vi "WS1050 36 DUT CP CV Sweep F12_B1_Ver1.2.vi"(0 "TMN DC\\CAP Data Log File Path":path=path "C:/WS1050 36 DUT Data", 1 "Test Program":string="WS1050 36 DUT CP CV Sweep SubVI", 3 "Lot#":string="WS1050", 4 "Wafer#":string="T7-EB", 5 "Board#":string="BRD5", 6 "Temp":string, 7 "error in (no error)":errorcluster, 8 "File Name":string="CYC_WS1050_T7_EB_65C_40V_25DC_EMPTY_BRD5_141017_1", 9 "Comment":string="CYC65C40V", 10 "Ke2400":refnum<visa-resource-name>="GPIB0::3::INSTR", 11 "PS1 Source":refnum<visa-resource-name>="GPIB0::5::INSTR", 12 "Serial Number":string[][](table)=[["DUT", "SN"], ["DUT1", "1"], ["DUT2", "2"], ["DUT3", "3"], ["DUT4", "4"], ["DUT5", "5"], ["DUT6", "6"], ["DUT7", "7"], ["DUT8", "8"], ["DUT9", "9"], ["DUT10", "10"], ["DUT11", "11"], ["DUT12", "12"], ["DUT13", "13"], ["DUT14", "14"], ["DUT15", "15"], ["DUT16", "16"], ["DUT17", "17"], ["DUT18", "18"], ["DUT19", "19"], ["DUT20", "20"], ["DUT21", "21"], ["DUT22", "22"], ["DUT23", "23"], ["DUT24", "24"], ["DUT25", "25"], ["DUT26", "26"], ["DUT27", "27"], ["DUT28", "28"], ["DUT29", "29"], ["DUT30", "30"], ["DUT31", "31"], ["DUT32", "32"], ["DUT33", "33"], ["DUT34", "34"], ["DUT35", "35"], ["DUT36", "36"]], 14 "CP Set to Run":dbl[][](array[numeric]), 16 "HD/Cycles Completed":string="Test Data", 18 "Ke2000":refnum<visa-resource-name>="GPIB0::9::INSTR") -> (13 "40V_1":string[][](table), 15 "40V_2":string[][](table), 17 "40V_3":string[][](table), 20 "Plot_1":dbl[][](graph) caption="(Y) Multi Plot 2", 21 "Plot_2":dbl[][](graph) caption="(Y) Multi Plot 2", 22 "Ke2400 Out":refnum<visa-resource-name>="GPIB0::3::INSTR", 23 "Plot_3":dbl[][](graph) caption="(Y) Multi Plot 2", 24 "CP Voltage":string, 25 "PS1 Out":refnum<visa-resource-name>, 26 "Ke2000 Out":refnum<visa-resource-name>="GPIB0::9::INSTR", 27 "error out":errorcluster)   [LabVIEW 2012]
uses:
  WS_VCAP Driver 029/Source/WSVCAP Shell/Type Defs/WSVCAP SHL I2C DUT Mask Mode Enum.ctl
panel:
  in  "Reg1_Bit Cntrl":string[](array[string])=["01", "02", "04", "08", "10", "20", "40", "80", "03", "06", "0C", "D8", "33", "66", "CC", "07", "0E", "1C", "38", "70", "E0", "0F", "1E", "3C", "78", "F0", "1F", "3E", "7C", "F8", "3F", "7E", "FC", "7F", "FE", "FD", "FB", "F7", "EF", "DF", "BF", "7F", "FC", "F9", "F3", "E7", "CF", "9F", "3F", "F8", "F1", "E3", "C7", "8F", "1F", "F0", "E1", "C3", "87", "0F", "E0", "C1", "83", "07", "C0", "81", "03", "AA", "55", "00"]
  out "date string":string="5/19/2014"
  in  "VPI_Cmd":string[](array[string])=["00", "3B", "00"]
  in  "VPI Name":string[](array[string])=["All_Drivers OFF", "All Drivers ON", "All Drivers OFF2"]
  in  "Tab Control":T1(tab)
  in  "Set VDD":dbl=3.7 format="%.3g"
  in  "Clock Rate (Hz)":dbl=1000000.0 caption="Meas Speed" format="%.1p Hz"
  out "AR  Measurent(Hz)":dbl
  in  "RFFE Slave Address":u8=7 caption="Slave Address" format="0x%02x"
  in  "CP VPI":i32(ring) items=["CP HDC 35V", "CP HDC 40.25V", "CP HDC 27.5V", "CP HDC 30.5V", "CP HDC 44V"]
  in  "Control Panel":T2={"CP C-V \nSweep"=TRUE, "HD/CYC"=FALSE, "E-CAL"=FALSE, "DVA"=FALSE, "VPI"=FALSE, "VSA"=FALSE, "HS"=FALSE}
  out "CP C-V Sweep":bool
  out "HD/CYC":bool
  out "E-CAL":bool
  out "DVA":bool
  out "VPI":bool
  out "VSA":bool
  out "HS":bool
  in  "Freq(Hz)":string="12K"
  in  "Test Sequences":i32(ring) items=["C1_C2_C3", "C2_C1_C3", "C3_C2_C1"]
  in  "WS1050/51":bool=TRUE
  in  "CP with DVA ON":i32(ring) items=["CP HDC 35V", "CP HDC 40.25V", "CP HDC 27.5V", "CP HDC 30.5V", "CP HDC 44V"]
  in  "% Duty Cycle":string="NA"
  in  "Cmin/Act":bool=TRUE
  in  "Current Input":string="71.772763E+0"
  out "NOM IDD OFF(uA)":string
  out "No of HD/Cycle\nCompleted":i32
  out "Loop \ncompleted":i32=1
  out "Previous Time":string="12:20:26 PM"
  out "STATUS":string="Idle...."
  out "Total Delta C2(pF)":string[](array[string])
  out "Total Delta C1(pF)":string[](array[string])
  out "Total Delta C3(pF)":string[](array[string])
  out "VPI C2":string[][](table)
  out "VPI C3":string[][](table)
  out "NOM IDD ON (uA)":string
  out "IDD_HD/CYC (uA)":string="164.601255E+0"
  out "IDD Stdby(uA)":string="2.606990E+0"
  out "VPI C1":string[][](table)
  out "Loops Run":i64
  out "VSA_V1":string[][](table)
  out "VSA_V2":string[][](table)
  out "VSA_V3":string[][](table)
  in  "VSA Voltage(V)":dbl[](array[numeric])=[-10.0, 0.0, 10.0]
  in  "X Repeat":i32=100
  out "% Delta C_T0":string[][](array[string])
  out "% Delta C":string[][](array[string])
  out "EFuse RB T0":string[](array[string])
  out "Current EFuse Read back":string[](array[string])
  out "EFuse Readback Status":bool[](array[boolean])
  in  "DeltaC Target Setting(pF)":dbl=7.375
  in  "Debug":bool
  in  "No of Rows\nFrom Spread Sheet":i32
  in  "Plot Delta Cmin":bool=TRUE
  in  "Plot":T3(ring)
  in  "Bank1":i32(ring)=6 items=["C1", "C2", "C3", "D_C1", "D_C2", "D_C3", "D_B1_C1", "D_B1_C2", "D_B1_C3"]
  in  "Bank2":i32(ring)=7 items=["C1", "C2", "C3", "D_C1", "D_C2", "D_C3", "D_B1_C1", "D_B1_C2", "D_B1_C3"]
  in  "Bank3":i32(ring)=8 items=["C1", "C2", "C3", "D_C1", "D_C2", "D_C3", "D_B1_C1", "D_B1_C2", "D_B1_C3"]
  # "Company:  WiSpry Inc\n20 Fairbanks Ste 198 Irvine CA 92618\n\nAuthor:  Andy V Tran\nCreated:  08/21/2015\nLabVIEW 2012 Pro\nTest Program:  WS1050 36 DUT CP CV Sweep SubVI\nFPGA: WS_VCAP Driver 029"
  # "Note for HD Duty Cycle:\n1.  Set time to start HD_DC (Min), default is 259200 (6 months) \n2.  Set Time for Duty Cycle ON/OFF, default setting is 2 minutes\n3.  No of Loops to RP = 3600s/(Time ALL ON(s) + Time ALL + OFF(s))\n4.  Set X Repeat = no of runs, default is 100 runs\n5.  Set TTF Completed to stop the test.\n\nVer 1.1 updated based on Ver1.0:\n1.  Updated the control panel ( CP C-V Sweep was set \"Yes\" by default)\n2.  CP Voltage sweep should be set up from look up table."
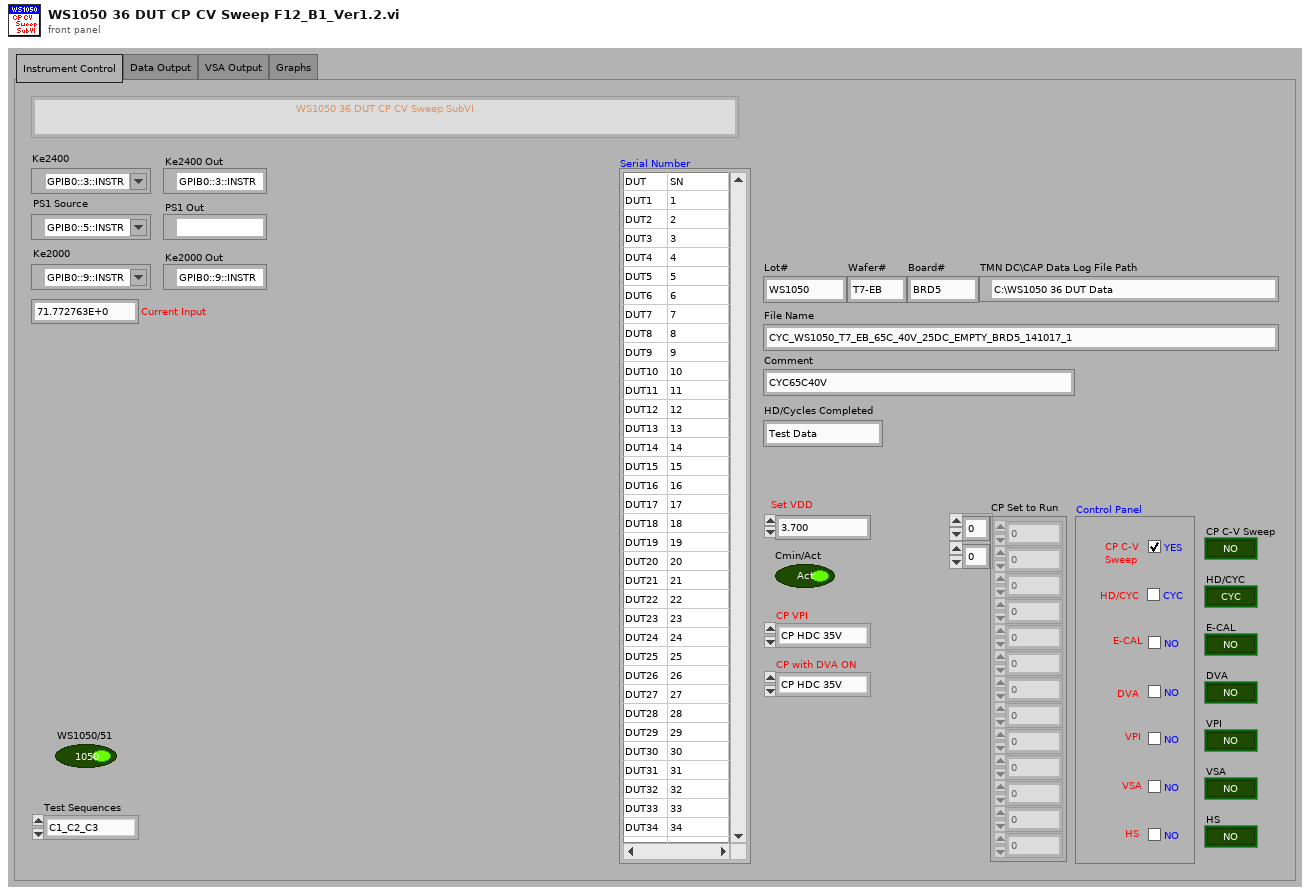
[diagram p1: front panel]
types:
  T1 = enum32{"Instrument Control", "Data Output", "VSA Output", "Graphs"}
  T2 = cluster{"CP C-V \nSweep":bool, "HD/CYC":bool, "E-CAL":bool, "DVA":bool, "VPI":bool, "VSA":bool, "HS":bool}
  T3 = enum16{"ALL DUTs", "DUT 01", "DUT 02", "DUT 03", "DUT 04", "DUT 05", "DUT 06", "DUT 07", "DUT 08", "DUT 09", "DUT 10", "DUT 11", "DUT 12", "DUT 13", "DUT 14", "DUT 15", "DUT 16", "DUT 17", "DUT 18", "DUT 19", "DUT 20", "DUT 21", "DUT 22", "DUT 23", "DUT 24", "DUT 25", "DUT 26", "DUT 27", "DUT 28", "DUT 29", "DUT 30", "DUT 31", "DUT 32", "DUT 33", "DUT 34", "DUT 35", "DUT 36"}
  T4 = typedef "WSVCAP SHL I2C DUT Mask Mode Enum.ctl" = enum16{"Custom", "C1", "C2", "C3", "All"}
  T5 = cluster{"Test Program ":string, "Comment":string, "Data Out":string, "Data Out":string, "CP Voltage":string, string, "% Duty Cycle":string, "CP Voltage":string, "string":string, "Freq(Hz)":string, "Board#":string}
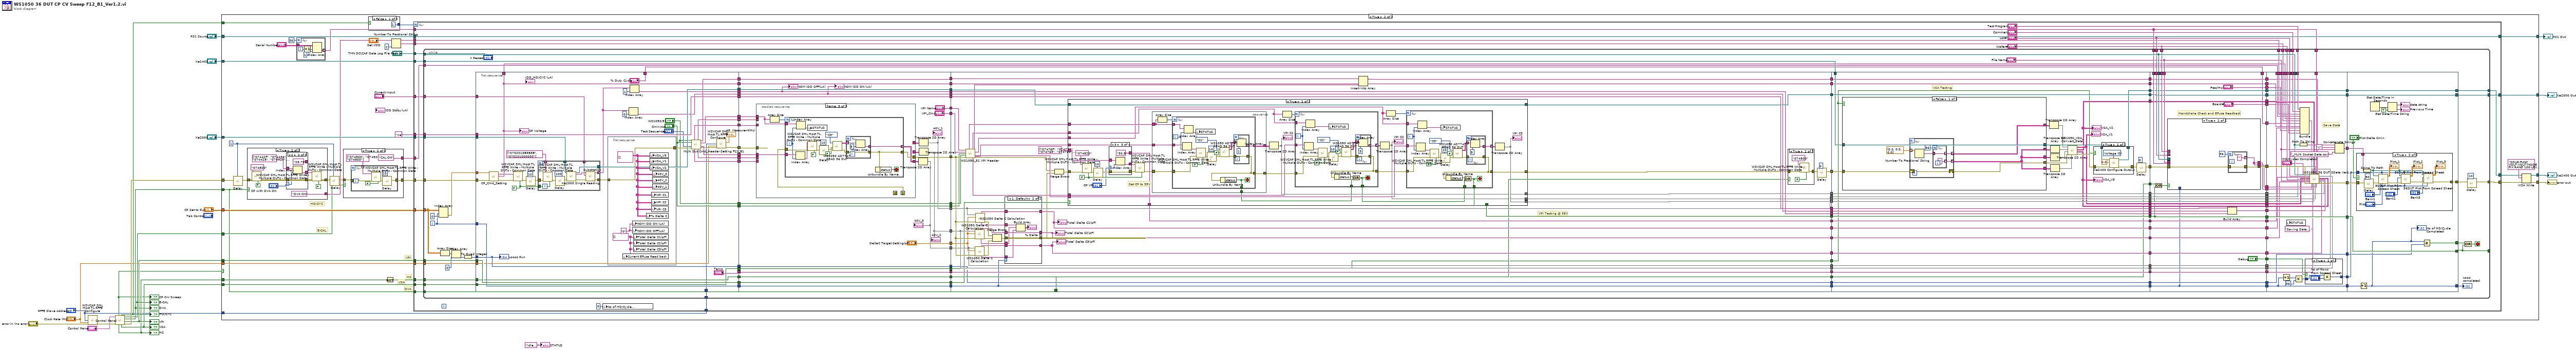
[diagram p0: block diagram]
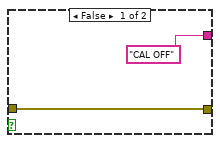
[diagram p3: hidden frame]
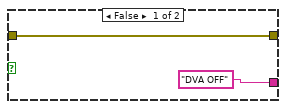
[diagram p4: hidden frame]
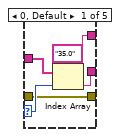
[diagram p5: hidden frame]
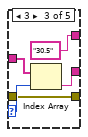
[diagram p6: hidden frame]
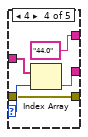
[diagram p7: hidden frame]
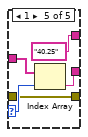
[diagram p8: hidden frame]
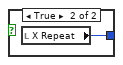
[diagram p9: hidden frame]
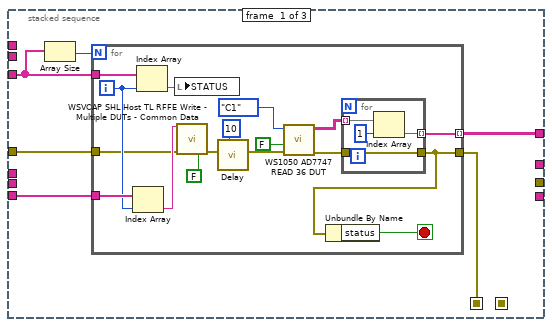
[diagram p10: hidden frame]
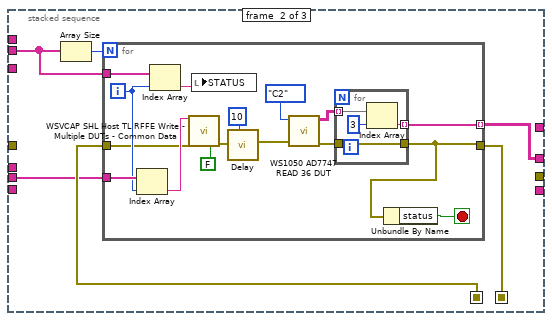
[diagram p11: hidden frame]
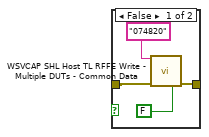
[diagram p12: hidden frame]
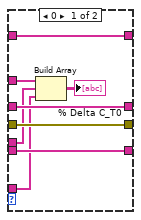
[diagram p13: hidden frame]
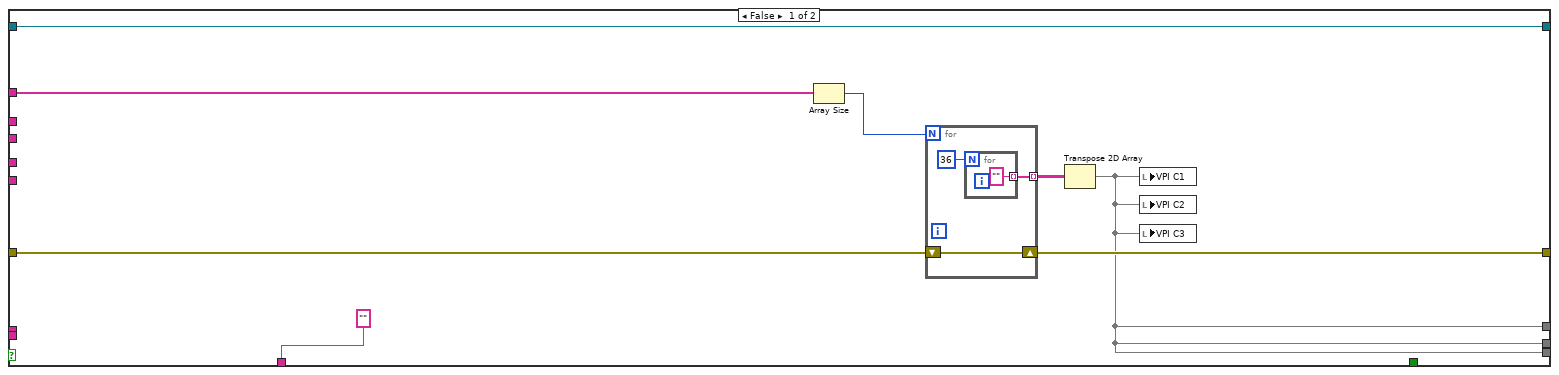
[diagram p14: hidden frame]
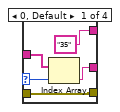
[diagram p15: hidden frame]
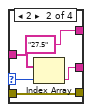
[diagram p16: hidden frame]
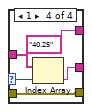
[diagram p17: hidden frame]
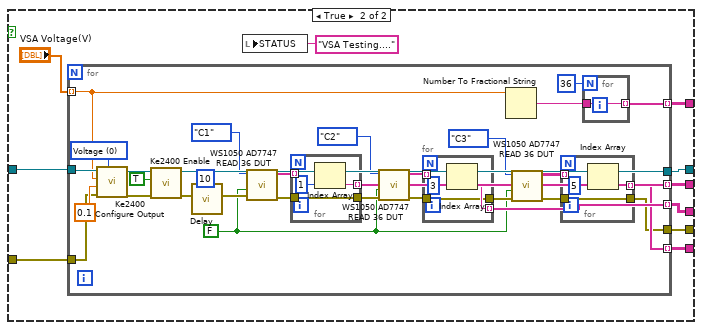
[diagram p19: hidden frame]
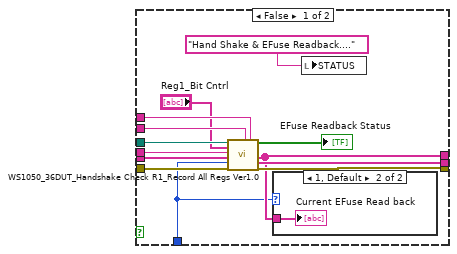
[diagram p20: hidden frame]
diagram:
  n1 = call "WSVCAP SHL Host TL RFFE Configure.vi"("RFFE Slave Address"="RFFE Slave Address", "Clock Rate (Hz)"="Clock Rate (Hz)", "error in"="error in (no error)") -> ("error out"=w4:errorcluster)  [unwired: 11 in, 1 out]
  n2 = call "Control Panel.vi"("error in (no error)"=w4, "Control Panel"="Control Panel") -> ("error out"=w12:errorcluster, "VPI"=w8:bool, "DVA"=w9:bool, "E-CAL"=w10:bool, "VSA"=w7:bool, "HD/CYC"=w11:bool, "HS"=w6:bool, "Verify Socket"=w1:bool)  [unwired: 2 in]
  "CP C-V Sweep" <- w1
  "E-CAL" <- w10
  "VPI" <- w8
  "VSA" <- w7
  "HS" <- w6
  "HD/CYC" <- w11
  "DVA" <- w9
  n3 = case shown="True" w1 {
    tunnel: w12 -> [w26 w29]
    tunnel: [w26 w34] -> w15
    tunnel: "CP Set to Run" -> [_ w64]
    tunnel: "PS1 Source" -> [w24 w31]
    tunnel: "Ke2000" -> [w25 w28]
    tunnel: [w25 w63] -> w22
    tunnel: [w24 w35] -> w21
    tunnel: "Ke2400" -> [w23 w61]
    tunnel: [w23 w58] -> w16
    tunnel: "RFFE Slave Address" -> [_ w56]
    tunnel: w11 -> [_ w41]
    tunnel: w10 -> [_ w40]
    tunnel: w9 -> [_ w30]
    tunnel: w8 -> [_ w39]
    tunnel: w7 -> [_ w38]
    tunnel: w6 -> [_ w37]
    tunnel: "Clock Rate (Hz)" -> [_ w33]
    frame False {
    }
    frame True {
      w32 = u32 1 ("milliseconds to wait")
      # "VSA"
      # "HS"
      # "HD/CYC"
      # "DVA"
      # "E-CAL"
      # "VPI"
      n4 = call "Delay.vi"("milliseconds to wait"=w32, "error in (no error)"=w29) -> ("error out"=w55:errorcluster)  [unwired: 9 in]
      n5 = case shown="True" w30 {
        tunnel: w55 -> [w82 w92]
        tunnel: [w82 w90] -> w53
        tunnel: ["DVA OFF" ("Data Out") "DVA ON" ("Data Out")] -> w54
        frame False {
        }
        frame True {
          n6 = call "WSVCAP SHL Host TL RFFE Write - Multiple DUTs - Common Data.vi"("Data Out"="074800", "error in"=w92, "Log (T)"=FALSE) -> ("error out"=w88:errorcluster)  [unwired: 12 in]
          n7 = case shown="2" "CP with DVA ON" {
            selector: "CP with DVA ON" -> [w98 w103 w108 w113 w117]
            tunnel: string[] ["07442F", "074436", "074428", "074429", "07443B"] -> [w99 w104 w109 w114 w119]
            tunnel: [w97 w102 w107 w112 w118] -> w84
            tunnel: ["35.0" ("Data Out") "29.75" ("Data Out") "30.5" ("Data Out") "44.0" ("Data Out") "40.25" ("Data Out")] -> _
            tunnel: w88 -> [w95 w100 w105 w110 w115]
            tunnel: [w95 w100 w105 w110 w115] -> w87
            frame 0, Default {
              n8 = Index Array(array=w99, index=w98) -> (element=w97:string)
            }
            frame 2 {
              n9 = Index Array(array=w104, index=w103) -> (element=w102:string)
            }
            frame 3 {
              n10 = Index Array(array=w109, index=w108) -> (element=w107:string)
            }
            frame 4 {
              n11 = Index Array(array=w114, index=w113) -> (element=w112:string)
            }
            frame 1 {
              n12 = Index Array(array=w119, index=w117) -> (element=w118:string)
            }
          }
          n13 = call "WSVCAP SHL Host TL RFFE Write - Multiple DUTs - Common Data.vi"("Data Out"=w84, "error in"=w87, "Log (T)"=FALSE) -> ("error out"=w90:errorcluster)  [unwired: 12 in]
        }
      }
      n14 = for {
        N: 36 -> [_]
        tunnel: "Serial Number" -> [w69]
        tunnel: [w67] -> w43 mode=indexing
        i -> [w66]
        n15 = Increment(x=w66) -> (x+1=w65:i32)
        n16 = Index Array(array=w69, index (row)=w65, index (col)=1 ("disabled index (col)")) -> (element=w67:string)
      }
      n17 = call "Delay.vi"("milliseconds to wait"=w32, "error in (no error)"=w53) -> ("error out"=w48:errorcluster)  [unwired: 9 in]
      n18 = case shown="True" w40 {
        tunnel: w48 -> [w70 w73]
        tunnel: [w70 w72] -> w47
        tunnel: ["CAL OFF" ("Data Out") "CAL ON" ("Data Out")] -> w49
        frame False {
        }
        frame True {
          n19 = for {
            tunnel: string[] ["074900", "074920", "074900"] -> [w81] mode=indexing
            tunnel: w73 -> [w78]
            tunnel: [w77] -> w72
            n20 = call "WSVCAP SHL Host TL RFFE Write - Multiple DUTs - Common Data.vi"("Data Out"=w81, "error in"=w78, "Log (T)"=FALSE) -> ("error out"=w80:errorcluster)  [unwired: 12 in]
            n21 = call "Delay.vi"("milliseconds to wait"=u32 10, "error in (no error)"=w80) -> ("error out"=w77:errorcluster)  [unwired: 9 in]
          }
        }
      }
      n22 = case shown="False" w41 {
        tunnel: [1 ("X Repeat") w121] -> w57
        frame False {
        }
        frame True {
          n23 = local read "X Repeat"() -> (w121:i32)
        }
      }
      n24 = Not(x=w37) -> (.not. x?=w42:bool)
      n25 = Number To Fractional String(number="Set VDD", precision (6)=i16 2) -> (F-format string=w51:string)  [unwired: 2 in]
      n26 = for {
        N: w57 -> [_]
        tunnel: w64 -> [w147]
        tunnel: [w143] -> w63
        tunnel: "na" ("In1 - In2") -> [w142]
        tunnel: w28 -> [w141]
        tunnel: "TMN DC\\CAP Data Log File Path" -> [w140]
        tunnel: w61 -> [w138]
        tunnel: [w137] -> w59
        tunnel: w31 -> [w124]
        tunnel: w56 -> [w135]
        tunnel: w54 -> [w134]
        tunnel: w51 -> [w133]
        tunnel: [w132] -> w50
        tunnel: w49 -> [w131]
        tunnel: w47 -> [w130]
        tunnel: w30 -> [w129]
        tunnel: w39 -> [w128]
        tunnel: w42 -> [w127]
        tunnel: w38 -> [w126]
        tunnel: w43 -> [w125]
        tunnel: [w124] -> w35
        tunnel: "Current Input" -> [w123]
        tunnel: w33 -> [w122]
        n27 = while {
          tunnel: w147 -> [w171]
          tunnel: w140 -> [w318]
          tunnel: "Lot#" -> [w317]
          tunnel: "Wafer#" -> [w316]
          tunnel: w125 -> [w315]
          tunnel: "Test Program" -> [w314]
          tunnel: w125 -> [w313]
          tunnel: "Comment" -> [w312]
          tunnel: "Lot#" -> [w311]
          tunnel: "Wafer#" -> [w310]
          tunnel: w141 -> [w307]
          tunnel: [w309] -> w143
          tunnel: w142 -> [w306]
          tunnel: w138 -> [w304]
          tunnel: [w303] -> w137
          tunnel: [w228] -> _
          tunnel: w135 -> [w227]
          tunnel: w134 -> [w210]
          tunnel: w133 -> [w209]
          tunnel: [w194] -> w132
          tunnel: w131 -> [w198]
          tunnel: w130 -> [w154]
          tunnel: w129 -> [w197]
          tunnel: w128 -> [w191]
          tunnel: w127 -> [w188]
          tunnel: w126 -> [w184]
          tunnel: w123 -> [w159]
          tunnel: w122 -> [w158]
          i -> [w172]
          stop <- w257 stop-if-true
          n28 = Index Array(array=w171, index (row)=w172, index (col)=0 ("disabled index (col)")) -> (element=w168:dbl)
          n29 = Array Size(array=w171) -> (size(s)=w170:i32[])
          n30 = Index Array(array=w170, index=0) -> (element=w161:i32)
          n31 = To Quad Integer(1:w161) -> (0:w160:i64)
          n32 = flat-sequence {
            tunnel: [w360] -> w302
            tunnel: w307 -> [w327]
            tunnel: w306 -> [w361]
            tunnel: [w361] -> w301
            tunnel: [w343] -> w300
            tunnel: [w340] -> w299
            tunnel: w154 -> [w326]
            tunnel: w172 -> [w328]
            tunnel: [w328] -> w256
            tunnel: ["Temp"] -> w251
            tunnel: [w347] -> w246
            tunnel: [w346] -> w245
            tunnel: [w345] -> w244
            tunnel: [w351] -> w234
            tunnel: [w348] -> w233
            tunnel: w227 -> [w319]
            tunnel: [w350] -> w218
            tunnel: [w349] -> w217
            tunnel: ["% Duty Cycle"] -> w208
            tunnel: [w325] -> w202
            tunnel: w191 -> [w357]
            tunnel: [w357] -> w190
            tunnel: w188 -> [w356]
            tunnel: [w356] -> w187
            tunnel: w184 -> [w355]
            tunnel: [w355] -> w183
            tunnel: [w322] -> w180
            tunnel: ["WS1050/51"] -> w177
            tunnel: ["Cmin/Act"] -> w175
            tunnel: w160 -> [w332]
            tunnel: w168 -> [w333]
            tunnel: [w332] -> w167
            tunnel: w159 -> [w331]
            tunnel: w158 -> [w320]
            tunnel: [w325] -> w155
            tunnel: w302 -> [w406]
            tunnel: w301 -> [w409]
            tunnel: w300 -> [w405]
            tunnel: w299 -> [w404]
            tunnel: [w399] -> w226
            tunnel: [w409] -> w225
            tunnel: [w405] -> w224
            tunnel: [w404] -> w223
            tunnel: w256 -> [w408]
            tunnel: [w408] -> w222
            tunnel: w251 -> [w407]
            tunnel: [w407] -> w221
            tunnel: [w406] -> w220
            tunnel: w246 -> [w403]
            tunnel: w245 -> [w386]
            tunnel: w244 -> [w387]
            tunnel: [w401] -> w219
            tunnel: w234 -> [w402]
            tunnel: w233 -> [w401]
            tunnel: w218 -> [w390]
            tunnel: w217 -> [w385]
            tunnel: [w400] -> w203
            tunnel: w202 -> [w400]
            tunnel: w190 -> [w398]
            tunnel: [w398] -> w189
            tunnel: w187 -> [w397]
            tunnel: [w397] -> w186
            tunnel: w183 -> [w396]
            tunnel: [w396] -> w182
            tunnel: w180 -> [w391]
            tunnel: w177 -> [w394]
            tunnel: [w394] -> w176
            tunnel: w175 -> [w393]
            tunnel: [w393] -> w174
            tunnel: w167 -> [w392]
            tunnel: [w392] -> w166
            tunnel: [w388] -> w153
            tunnel: [w384] -> w152
            tunnel: [w382] -> w151
            tunnel: ["DeltaC Target Setting(pF)"] -> w150
            tunnel: ["VPI Name"] -> w149
            tunnel: ["VPI_Cmd"] -> w148
            tunnel: [w544] -> w298
            tunnel: [w513] -> w297
            tunnel: [w533] -> w296
            tunnel: [w524] -> w295
            tunnel: [w546] -> w294
            tunnel: [w545] -> w293
            tunnel: [w543] -> w292
            tunnel: [w539] -> w291
            tunnel: [w538] -> w290
            tunnel: [w534] -> w255
            tunnel: [w542] -> w250
            tunnel: [w540] -> w247
            tunnel: [w537] -> w243
            tunnel: [w535] -> w242
            tunnel: [w532] -> w237
            tunnel: [w521] -> w232
            tunnel: [w520] -> w231
            tunnel: [w519] -> w230
            tunnel: [w518] -> w204
            tunnel: [w517] -> w201
            tunnel: [w510] -> w185
            tunnel: [w509] -> w181
            tunnel: [w496] -> w165
            tunnel: w150 -> [w530]
            tunnel: w151 -> [w524]
            tunnel: w152 -> [w531]
            tunnel: w226 -> [w533]
            tunnel: w225 -> [w543]
            tunnel: w224 -> [w539]
            tunnel: w223 -> [w538]
            tunnel: w222 -> [w534]
            tunnel: w221 -> [w542]
            tunnel: w220 -> [w541]
            tunnel: w219 -> [w536]
            tunnel: w203 -> [w518]
            tunnel: w189 -> [w511]
            tunnel: w186 -> [w510]
            tunnel: w182 -> [w509]
            tunnel: w176 -> [w508]
            tunnel: w174 -> [w497]
            tunnel: w166 -> [w496]
            tunnel: w153 -> [w532]
            tunnel: w197 -> [w516]
            tunnel: w149 -> [w492]
            tunnel: w148 -> [w491]
            tunnel: w298 -> [w751]
            tunnel: [w751] -> w289
            tunnel: [w737] -> w288
            tunnel: [w750] -> w287
            tunnel: w297 -> [w749]
            tunnel: w296 -> [w748]
            tunnel: w295 -> [w747]
            tunnel: [w748] -> w286
            tunnel: [w747] -> w285
            tunnel: w294 -> [w746]
            tunnel: [w746] -> w284
            tunnel: w293 -> [w745]
            tunnel: [w745] -> w283
            tunnel: w292 -> [w744]
            tunnel: [w744] -> w282
            tunnel: w291 -> [w743]
            tunnel: [w743] -> w281
            tunnel: w290 -> [w742]
            tunnel: [w742] -> w280
            tunnel: w304 -> [w741]
            tunnel: [w739] -> w279
            tunnel: [w719] -> w278
            tunnel: [w720] -> w277
            tunnel: [w718] -> w276
            tunnel: w255 -> [w735]
            tunnel: [w735] -> w254
            tunnel: w250 -> [w734]
            tunnel: [w734] -> w249
            tunnel: w247 -> [w750]
            tunnel: w243 -> [w732]
            tunnel: w242 -> [w733]
            tunnel: [w733] -> w241
            tunnel: [w732] -> w239
            tunnel: w237 -> [w731]
            tunnel: [w731] -> w236
            tunnel: w232 -> [w717]
            tunnel: w231 -> [w716]
            tunnel: w230 -> [w715]
            tunnel: [w712] -> w229
            tunnel: [w717] -> w216
            tunnel: [w716] -> w214
            tunnel: [w715] -> w212
            tunnel: [w714] -> w205
            tunnel: w204 -> [w714]
            tunnel: w201 -> [w713]
            tunnel: [w713] -> w200
            tunnel: w185 -> [w712]
            tunnel: w181 -> [w711]
            tunnel: w165 -> [w710]
            tunnel: [w710] -> w164
            tunnel: w289 -> [w845]
            tunnel: [w845] -> w275
            tunnel: w288 -> [w866]
            tunnel: [w865] -> w274
            tunnel: w318 -> [w867]
            tunnel: w317 -> [w864]
            tunnel: w316 -> [w863]
            tunnel: w315 -> [w862]
            tunnel: [w861] -> w273
            tunnel: w287 -> [w855]
            tunnel: [w855] -> w272
            tunnel: w286 -> [w860]
            tunnel: w285 -> [w859]
            tunnel: [w860] -> w271
            tunnel: [w859] -> w270
            tunnel: [w853] -> w269
            tunnel: w284 -> [w858]
            tunnel: [w858] -> w268
            tunnel: w283 -> [w857]
            tunnel: [w857] -> w267
            tunnel: [w856] -> w266
            tunnel: w282 -> [w854]
            tunnel: w281 -> [w852]
            tunnel: w280 -> [w851]
            tunnel: "File Name" -> [w850]
            tunnel: w279 -> [w849]
            tunnel: [w849] -> w265
            tunnel: w278 -> [w848]
            tunnel: [w848] -> w264
            tunnel: [w847] -> w263
            tunnel: w277 -> [w847]
            tunnel: w276 -> [w846]
            tunnel: [w846] -> w262
            tunnel: w254 -> [w829]
            tunnel: [w829] -> w252
            tunnel: w249 -> [w843]
            tunnel: [w843] -> w248
            tunnel: w241 -> [w842]
            tunnel: [w842] -> w240
            tunnel: w239 -> [w841]
            tunnel: [w841] -> w238
            tunnel: w236 -> [w840]
            tunnel: [w840] -> w235
            tunnel: w229 -> [w839]
            tunnel: w216 -> [w838]
            tunnel: [w838] -> w215
            tunnel: w214 -> [w837]
            tunnel: [w837] -> w213
            tunnel: w212 -> [w836]
            tunnel: [w836] -> w211
            tunnel: w208 -> [w835]
            tunnel: [w835] -> w207
            tunnel: [w834] -> w206
            tunnel: w205 -> [w834]
            tunnel: w200 -> [w833]
            tunnel: [w833] -> w199
            tunnel: ["Freq(Hz)"] -> w179
            tunnel: ["Board#"] -> w178
            tunnel: w164 -> [w830]
            tunnel: [w830] -> w163
            tunnel: ["Debug"] -> w157
            tunnel: w275 -> [w940]
            tunnel: w274 -> [w939]
            tunnel: w318 -> [w906]
            tunnel: w314 -> [w934]
            tunnel: w313 -> [w937]
            tunnel: w312 -> [w933]
            tunnel: w311 -> [w936]
            tunnel: w310 -> [w932]
            tunnel: w273 -> [w935]
            tunnel: [w940] -> w259
            tunnel: [w938] -> w260
            tunnel: w272 -> [w930]
            tunnel: [w930] -> w261
            tunnel: w271 -> [w929]
            tunnel: w270 -> [w917]
            tunnel: w269 -> [w928]
            tunnel: w268 -> [w927]
            tunnel: w267 -> [w919]
            tunnel: w266 -> [w926]
            tunnel: "File Name" -> [w900]
            tunnel: w265 -> [w925]
            tunnel: [w925] -> w258
            tunnel: w264 -> [w924]
            tunnel: w263 -> [w923]
            tunnel: w262 -> [w922]
            tunnel: [w902] -> w253
            tunnel: w252 -> [w902]
            tunnel: w248 -> [w921]
            tunnel: w240 -> [w920]
            tunnel: w238 -> [w918]
            tunnel: w235 -> [w889]
            tunnel: w215 -> [w916]
            tunnel: w213 -> [w915]
            tunnel: w211 -> [w914]
            tunnel: w210 -> [w913]
            tunnel: w198 -> [w912]
            tunnel: w155 -> [w911]
            tunnel: w209 -> [w910]
            tunnel: w207 -> [w909]
            tunnel: w206 -> [w908]
            tunnel: w199 -> [w907]
            tunnel: [w904] -> w196
            tunnel: [w897] -> w192
            tunnel: w179 -> [w896]
            tunnel: w178 -> [w894]
            tunnel: w163 -> [w893]
            tunnel: [w893] -> w162
            tunnel: w157 -> [w891]
            tunnel: [w958] -> w308
            tunnel: [w959] -> w309
            tunnel: [w960] -> w228
            tunnel: w261 -> [w959]
            tunnel: w260 -> [w952]
            tunnel: w259 -> [w960]
            tunnel: w258 -> [w953]
            tunnel: [w953] -> w303
            tunnel: w253 -> [w946]
            tunnel: [w951] -> w193
            tunnel: w196 -> [w950]
            tunnel: w192 -> [w948]
            tunnel: w162 -> [w947]
            tunnel: [w945] -> w156
            frame #0 {
              w354 = FALSE ("Log (T)")
              n33 = call "CP_Cmd_Setting.vi"("error in (no error)"=w326, "Input"=w333) -> ("error out"=w335:errorcluster, "CP Voltage"=w325:string, "Send Cmd"=w334:string)  [unwired: 6 in, 1 out]
              "CP Voltage" <- w325
              n34 = call "WSVCAP SHL Host TL RFFE Write - Multiple DUTs - Common Data.vi"("Data Out"=w334, "error in"=w335, "Log (T)"=w354) -> ("error out"=w358:errorcluster)  [unwired: 12 in]
              n35 = call "Delay.vi"("milliseconds to wait"=u32 10, "error in (no error)"=w358) -> ("error out"=w338:errorcluster)  [unwired: 9 in]
              n36 = for {
                tunnel: [w374] -> w360
                tunnel: [w373] -> w324
                tunnel: w354 -> [w372]
                tunnel: w327 -> [w371]
                tunnel: w338 -> [w367]
                tunnel: string[] ["0702013B3B3B", "070201000000"] -> [w364] mode=indexing
                tunnel: [w363] -> w341 mode=indexing
                tunnel: w331 -> [w362]
                n37 = call "WSVCAP SHL Host TL RFFE Write - Multiple DUTs - Common Data.vi"("Data Out"=w364, "error in"=w367, "Log (T)"=w372) -> ("error out"=w368:errorcluster)  [unwired: 12 in]
                n38 = call "Delay.vi"("milliseconds to wait"=u32 100, "error in (no error)"=w368) -> ("error out"=w369:errorcluster)  [unwired: 9 in]
                n39 = call "Ke2000 Single Reading.vi"("error in (no error)"=w369, "VISA resource name"=w371) -> ("error out"=w366:errorcluster, "VISA resource name out"=w374:refnum<visa-resource-name>, "uA"=w365:string)  [unwired: 5 in, 2 out]
                n40 = call "Substration.vi"("error in (no error)"=w366, "Input2"=w362, "Input1"=w365) -> ("error out"=w373:errorcluster, "In1 - In2"=w363:string)  [unwired: 7 in]
              }
              n41 = flat-sequence {
                tunnel: [w375] -> w353
                tunnel: w324 -> [w375]
                frame #0 {
                  w376 = "0" ("NOM IDD OFF(uA)")
                  w377 = string[] []
                  w378 = string[][] []
                  n42 = local write "Current EFuse Read back"(w377) -> ()
                  n43 = local write "NOM IDD ON (uA)"(w376) -> ()
                  n44 = local write "NOM IDD OFF(uA)"(w376) -> ()
                  n45 = local write "Total Delta C1(pF)"(w377) -> ()
                  n46 = local write "Total Delta C2(pF)"(w377) -> ()
                  n47 = local write "Total Delta C3(pF)"(w377) -> ()
                  n48 = local write "% Delta C"(w378) -> ()
                  n49 = local write "VSA_V3"(w378) -> ()
                  n50 = local write "VSA_V1"(w378) -> ()
                  n51 = local write "VSA_V2"(w378) -> ()
                  n52 = local write "VPI C1"(w378) -> ()
                  n53 = local write "VPI C2"(w378) -> ()
                  n54 = local write "VPI C3"(w378) -> ()
                  n55 = local write "40V_3"(w378) -> ()
                  n56 = local write "40V_2"(w378) -> ()
                  n57 = local write "40V_1"(w378) -> ()
                }
              }
              n58 = Index Array(array=w341, index=0) -> (element=w343:string)
              n59 = Index Array(array=w341, index=1) -> (element=w340:string)
              n60 = call "Multi Dut Cmd_Header Setting F12_B1.vi"("WS1050/51"="WS1050/51", "Cmin/Act"="Cmin/Act", "Test Seq"="Test Sequences", "error in (no error)"=w353) -> ("Name 1"=w351:string[], "Name 2"=w350:string[], "Name Header"=w348:string[], "Name 3"=w349:string[], "Cmd 3"=w345:string[], "Cmd 1"=w347:string[], "Cmd 2"=w346:string[], "error out"=w321:errorcluster)  [unwired: 2 in, 2 out]
              n61 = call "WSVCAP SHL Host TL RFFE Configure.vi"("RFFE Slave Address"=w319, "Clock Rate (Hz)"=w320, "error in"=w321) -> ("Actual Rate (Hz)"=→"AR  Measurent(Hz)":dbl, "error out"=w322:errorcluster)  [unwired: 11 in]
              "Loops Run" <- w332
            }
            frame #1 {
              n62 = stacked-sequence {
                seq-local: [w410 _ _] -> [_ w442 _]
                seq-local: [_ w439 _] -> [_ _ w468]
                tunnel: w403 -> [w415 _ _]
                tunnel: w402 -> [w411 _ _]
                tunnel: w391 -> [w414 _ _]
                tunnel: [w413 _ _] -> w395
                tunnel: w390 -> [_ w440 _]
                tunnel: [_ w438 _] -> w389
                tunnel: w387 -> [_ _ w467]
                tunnel: w386 -> [_ w437 _]
                tunnel: w385 -> [_ _ w465]
                tunnel: [_ _ w464] -> w384
                tunnel: [_ _ w463] -> w383
                frame #0 {
                  n63 = Array Size(array=w411) -> (size(s)=w412:i32)
                  n64 = for {
                    N: w412 -> [_]
                    tunnel: w415 -> [w432]
                    tunnel: [w428] -> w413 mode=indexing
                    tunnel: w411 -> [w430]
                    tunnel: w414 -> [w419]
                    tunnel: [w420] -> w410
                    i -> [w427]
                    stop <- w417 stop-if-true
                    n65 = Index Array(array=w432, index=w427) -> (element=w431:string)
                    n66 = Index Array(array=w430, index=w427) -> (element=w429:string)
                    n67 = local write "STATUS"(w429) -> ()
                    n68 = call "WSVCAP SHL Host TL RFFE Write - Multiple DUTs - Common Data.vi"("Data Out"=w431, "error in"=w419, "Log (T)"=FALSE) -> ("error out"=w422:errorcluster)  [unwired: 12 in]
                    n69 = call "Delay.vi"("milliseconds to wait"=u32 10, "error in (no error)"=w422) -> ("error out"=w426:errorcluster)  [unwired: 9 in]
                    n70 = call "WS1050 AD7747 READ 36 DUT.vi"("error in"=w426, "Log (T)"=FALSE, "DUT Mask Mode (All)"=WSVCAP_SHL_I2C_DUT_Mask_Mode_Enum."C1") -> ("error out"=w424:errorcluster, "AD7747 Values"=w425:string[][])  [unwired: 7 in]
                    n71 = for {
                      tunnel: w425 -> [w435] mode=indexing
                      tunnel: w424 -> [w436]
                      tunnel: [w436] -> w420
                      tunnel: [w433] -> w428 mode=indexing
                      n72 = Index Array(array=w435, index=1) -> (element=w433:string)
                    }
                    n73 = Unbundle By Name(w420) -> ("status"=w417:bool)
                  }
                }
                frame #1 {
                  n74 = Array Size(array=w440) -> (size(s)=w441:i32)
                  n75 = for {
                    N: w441 -> [_]
                    tunnel: w437 -> [w458]
                    tunnel: [w454] -> w438 mode=indexing
                    tunnel: w440 -> [w456]
                    tunnel: w442 -> [w445]
                    tunnel: [w446] -> w439
                    i -> [w453]
                    stop <- w443 stop-if-true
                    n76 = Index Array(array=w458, index=w453) -> (element=w457:string)
                    n77 = Index Array(array=w456, index=w453) -> (element=w455:string)
                    n78 = call "WSVCAP SHL Host TL RFFE Write - Multiple DUTs - Common Data.vi"("Data Out"=w457, "error in"=w445, "Log (T)"=FALSE) -> ("error out"=w448:errorcluster)  [unwired: 12 in]
                    n79 = local write "STATUS"(w455) -> ()
                    n80 = call "Delay.vi"("milliseconds to wait"=u32 10, "error in (no error)"=w448) -> ("error out"=w452:errorcluster)  [unwired: 9 in]
                    n81 = call "WS1050 AD7747 READ 36 DUT.vi"("error in"=w452, "DUT Mask Mode (All)"=WSVCAP_SHL_I2C_DUT_Mask_Mode_Enum."C2") -> ("error out"=w450:errorcluster, "AD7747 Values"=w451:string[][])  [unwired: 8 in]
                    n82 = for {
                      tunnel: w451 -> [w461] mode=indexing
                      tunnel: w450 -> [w462]
                      tunnel: [w462] -> w446
                      tunnel: [w459] -> w454 mode=indexing
                      n83 = Index Array(array=w461, index=3) -> (element=w459:string)
                    }
                    n84 = Unbundle By Name(w446) -> ("status"=w443:bool)
                  }
                }
                frame #2 {
                  n85 = Array Size(array=w465) -> (size(s)=w466:i32)
                  n86 = for {
                    N: w466 -> [_]
                    tunnel: w467 -> [w485]
                    tunnel: [w481] -> w463 mode=indexing
                    tunnel: w465 -> [w483]
                    tunnel: w468 -> [w472]
                    tunnel: [w473] -> w464
                    i -> [w480]
                    stop <- w470 stop-if-true
                    n87 = Index Array(array=w485, index=w480) -> (element=w484:string)
                    n88 = Index Array(array=w483, index=w480) -> (element=w482:string)
                    n89 = local write "STATUS"(w482) -> ()
                    n90 = call "WSVCAP SHL Host TL RFFE Write - Multiple DUTs - Common Data.vi"("Data Out"=w484, "error in"=w472, "Log (T)"=FALSE) -> ("error out"=w475:errorcluster)  [unwired: 12 in]
                    n91 = call "Delay.vi"("milliseconds to wait"=u32 10, "error in (no error)"=w475) -> ("error out"=w479:errorcluster)  [unwired: 9 in]
                    n92 = call "WS1050 AD7747 READ 36 DUT.vi"("error in"=w479, "Log (T)"=FALSE, "DUT Mask Mode (All)"=WSVCAP_SHL_I2C_DUT_Mask_Mode_Enum."C3") -> ("error out"=w477:errorcluster, "AD7747 Values"=w478:string[][])  [unwired: 7 in]
                    n93 = for {
                      tunnel: w478 -> [w488] mode=indexing
                      tunnel: w477 -> [w489]
                      tunnel: [w489] -> w473
                      tunnel: [w486] -> w481 mode=indexing
                      n94 = Index Array(array=w488, index=5) -> (element=w486:string)
                    }
                    n95 = Unbundle By Name(w473) -> ("status"=w470:bool)
                  }
                }
              }
              n96 = Transpose 2D Array(2D array=w383) -> (transposed array=w382:string[][])
              "40V_3" <- w382
              n97 = Transpose 2D Array(2D array=w395) -> (transposed array=w399:string[][])
              "40V_1" <- w399
              n98 = Transpose 2D Array(2D array=w389) -> (transposed array=w388:string[][])
              "40V_2" <- w388
              "NOM IDD ON (uA)" <- w405
              "NOM IDD OFF(uA)" <- w404
            }
            frame #2 {
              # "VPI Testing @ 35V"
              n99 = call "WS1050_51 VPI Header.vi"("VPI Name"=w492, "VPI_Cmd"=w491, "Cmin/Act"=w497, "WS1050/51"=w508, "error in (no error)"=w531) -> ("VPI_1"=w507:string[], "VPI_2"=w505:string[], "VPI Header"=w506:string[], "VPI_3"=w504:string[], "Cmd_3"=w501:string[], "Cmd_1"=w503:string[], "Cmd_2"=w502:string[], "error out"=w500:errorcluster)  [unwired: 3 in]
              n100 = call "WS1050 Delta C Calculation.vi"("error in (no error)"=w531, "DCap Target(pF)"=w530, "Input"=w532) -> ("error out"=w529:errorcluster, "% Bank DeltaC"=w523:string[], "Delta B1(pF)"=w494:string[])  [unwired: 3 in, 3 out]
              n101 = call "WS1050 Delta C Calculation.vi"("error in (no error)"=w531, "DCap Target(pF)"=w530, "Input"=w524) -> ("error out"=w527:errorcluster, "% Bank DeltaC"=w522:string[], "Delta B1(pF)"=w493:string[])  [unwired: 3 in, 3 out]
              n102 = call "WS1050 Delta C Calculation.vi"("error in (no error)"=w531, "DCap Target(pF)"=w530, "Input"=w533) -> ("error out"=w528:errorcluster, "% Bank DeltaC"=w525:string[], "Delta B1(pF)"=w495:string[])  [unwired: 3 in, 3 out]
              n103 = Merge Errors(w528, w529, w527) -> (w526:errorcluster)
              n104 = case shown="1, Default" w534 {
                tunnel: w526 -> [w562 w570]
                tunnel: [w562 w570] -> w499
                tunnel: w525 -> [w558 w566]
                tunnel: w523 -> [w557 w565]
                tunnel: w522 -> [w556 w564]
                tunnel: w495 -> [w561 w569]
                tunnel: [w561 w569] -> w521
                tunnel: w494 -> [w560 w568]
                tunnel: [w560 w568] -> w520
                tunnel: w493 -> [w559 w567]
                tunnel: [w559 w567] -> w519
                frame 0 {
                  n105 = Build Array(w558, w557, w556) -> (→"% Delta C_T0":string[][])
                }
                frame 1, Default {
                  n106 = Build Array(w566, w565, w564) -> (→"% Delta C":string[][])
                }
              }
              "Total Delta C1(pF)" <- w521
              "Total Delta C2(pF)" <- w520
              "Total Delta C3(pF)" <- w519
              n107 = Merge Errors(w500, w499) -> (w498:errorcluster)
              n108 = case shown="True" w511 {
                tunnel: [w573 w592] -> w515
                tunnel: [w571 w615] -> w546
                tunnel: [w571 w600] -> w545
                tunnel: [_ w598] -> w544
                tunnel: w541 -> [w578 w614]
                tunnel: [w578 w614] -> w540
                tunnel: w503 -> [_ w613]
                tunnel: w502 -> [_ w607]
                tunnel: w501 -> [_ w602]
                tunnel: [w571 w612] -> w537
                tunnel: w507 -> [w576 w610]
                tunnel: w505 -> [_ w608]
                tunnel: w504 -> [_ w603]
                tunnel: ["" ("string") w597] -> w517
                tunnel: w498 -> [w574 w590]
                tunnel: string[] ["07476F", "074776", "074765", "074769", "07477B"] -> [_ w583]
                frame False {
                  n109 = Array Size(array=w576) -> (size(s)=w575:i32)
                  n110 = for {
                    N: w575 -> [_]
                    tunnel: [w580] -> w572 mode=indexing
                    shift-right: [w579] -> w573
                    shift-left: w574 -> [w579]
                    n111 = for {
                      N: 36 -> [_]
                      tunnel: [""] -> w580 mode=indexing
                    }
                  }
                  n112 = Transpose 2D Array(2D array=w572) -> (transposed array=w571:string[][])
                  n113 = local write "VPI C1"(w571) -> ()
                  n114 = local write "VPI C2"(w571) -> ()
                  n115 = local write "VPI C3"(w571) -> ()
                }
                frame True {
                  w591 = FALSE ("Log (T)")
                  # "Set CP to 35V"
                  n116 = call "WSVCAP SHL Host TL RFFE Write - Multiple DUTs - Common Data.vi"("Data Out"="074820", "error in"=w590, "Log (T)"=w591) -> ("error out"=w588:errorcluster)  [unwired: 12 in]
                  n117 = call "Delay.vi"("milliseconds to wait"=u32 10, "error in (no error)"=w588) -> ("error out"=w593:errorcluster)  [unwired: 9 in]
                  n118 = case shown="3" "CP VPI" {
                    selector: "CP VPI" -> [w647 w652 w657 w661]
                    tunnel: w583 -> [w648 w653 w658 w663]
                    tunnel: [w646 w651 w656 w662] -> w586
                    tunnel: [w644 w649 w654 w659] -> w585
                    tunnel: ["35" ("string") "27.5" ("string") "30.5" ("string") "40.25" ("string")] -> w597
                    tunnel: w593 -> [w644 w649 w654 w659]
                    frame 0, Default {
                      n119 = Index Array(array=w648, index=w647) -> (element=w646:string)
                    }
                    frame 2 {
                      n120 = Index Array(array=w653, index=w652) -> (element=w651:string)
                    }
                    frame 3 {
                      n121 = Index Array(array=w658, index=w657) -> (element=w656:string)
                    }
                    frame 1 {
                      n122 = Index Array(array=w663, index=w661) -> (element=w662:string)
                    }
                  }
                  n123 = call "WSVCAP SHL Host TL RFFE Write - Multiple DUTs - Common Data.vi"("Data Out"=w586, "error in"=w585, "Log (T)"=w591) -> ("error out"=w596:errorcluster)  [unwired: 12 in]
                  n124 = stacked-sequence {
                    tunnel: w613 -> [w621]
                    tunnel: [w620] -> w611
                    tunnel: w610 -> [w619]
                    tunnel: [w618] -> w606
                    tunnel: w596 -> [w617]
                    tunnel: [w616] -> w595
                    frame #0 {
                      n125 = Array Size(array=w619) -> (size(s)=w622:i32)
                      n126 = for {
                        N: w622 -> [_]
                        tunnel: w621 -> [w639]
                        tunnel: [w623] -> w618
                        tunnel: [w637] -> w620 mode=indexing
                        tunnel: w619 -> [w636]
                        tunnel: w617 -> [w625]
                        tunnel: [w627] -> w616
                        i -> [w635]
                        stop <- w623 stop-if-true
                        n127 = Index Array(array=w639, index=w635) -> (element=w638:string)
                        n128 = Index Array(array=w636, index=w635) -> (element=w634:string)
                        n129 = local write "STATUS"(w634) -> ()
                        n130 = call "WSVCAP SHL Host TL RFFE Write - Multiple DUTs - Common Data.vi"("Data Out"=w638, "error in"=w625, "Log (T)"=FALSE) -> ("error out"=w633:errorcluster)  [unwired: 12 in]
                        n131 = call "Delay.vi"("milliseconds to wait"=u32 10, "error in (no error)"=w633) -> ("error out"=w629:errorcluster)  [unwired: 9 in]
                        n132 = call "WS1050 AD7747 READ 36 DUT.vi"("error in"=w629, "Log (T)"=FALSE, "DUT Mask Mode (All)"=WSVCAP_SHL_I2C_DUT_Mask_Mode_Enum."C1") -> ("error out"=w631:errorcluster, "AD7747 Values"=w630:string[][])  [unwired: 7 in]
                        n133 = for {
                          tunnel: [w642] -> w637 mode=indexing
                          tunnel: w631 -> [w641]
                          tunnel: [w641] -> w627
                          tunnel: w630 -> [w640] mode=indexing
                          n134 = Index Array(array=w640, index=1) -> (element=w642:string)
                        }
                        n135 = Unbundle By Name(w627) -> ("status"=w623:bool)
                      }
                    }
                  }
                  n136 = Transpose 2D Array(2D array=w611) -> (transposed array=w615:string[][])
                  "VPI C1" <- w615
                  n137 = Array Size(array=w608) -> (size(s)=w609:i32)
                  n138 = for {
                    N: w609 -> [_]
                    tunnel: w607 -> [w705]
                    tunnel: w606 -> [w703]
                    tunnel: [w702] -> w599
                    tunnel: [w700] -> w605 mode=indexing
                    tunnel: w608 -> [w699]
                    tunnel: w595 -> [w688]
                    tunnel: [w690] -> w594
                    i -> [w698]
                    stop <- w702 stop-if-true
                    n139 = Index Array(array=w705, index=w698) -> (element=w701:string)
                    n140 = Index Array(array=w699, index=w698) -> (element=w697:string)
                    n141 = call "WSVCAP SHL Host TL RFFE Write - Multiple DUTs - Common Data.vi"("Data Out"=w701, "error in"=w688, "Log (T)"=FALSE) -> ("error out"=w696:errorcluster)  [unwired: 12 in]
                    n142 = local write "STATUS"(w697) -> ()
                    n143 = call "Delay.vi"("milliseconds to wait"=u32 10, "error in (no error)"=w696) -> ("error out"=w692:errorcluster)  [unwired: 9 in]
                    n144 = call "WS1050 AD7747 READ 36 DUT.vi"("error in"=w692, "Log (T)"=FALSE, "DUT Mask Mode (All)"=WSVCAP_SHL_I2C_DUT_Mask_Mode_Enum."C2") -> ("error out"=w694:errorcluster, "AD7747 Values"=w693:string[][])  [unwired: 7 in]
                    n145 = for {
                      tunnel: [w708] -> w700 mode=indexing
                      tunnel: w694 -> [w707]
                      tunnel: [w707] -> w690
                      tunnel: w693 -> [w706] mode=indexing
                      n146 = Index Array(array=w706, index=3) -> (element=w708:string)
                    }
                    n147 = Unbundle By Name(w690) -> ("status"=w704:bool)
                    n148 = Or(x=w704, y=w703) -> (x .or. y?=w702:bool)
                  }
                  n149 = Transpose 2D Array(2D array=w605) -> (transposed array=w612:string[][])
                  "VPI C2" <- w612
                  n150 = Array Size(array=w603) -> (size(s)=w604:i32)
                  n151 = for {
                    N: w604 -> [_]
                    tunnel: w602 -> [w682]
                    tunnel: w599 -> [w680]
                    tunnel: [w679] -> w598
                    tunnel: [w677] -> w601 mode=indexing
                    tunnel: w603 -> [w676]
                    tunnel: w594 -> [w665]
                    tunnel: [w667] -> w592
                    i -> [w675]
                    stop <- w679 stop-if-true
                    n152 = Index Array(array=w682, index=w675) -> (element=w678:string)
                    n153 = Index Array(array=w676, index=w675) -> (element=w674:string)
                    n154 = call "WSVCAP SHL Host TL RFFE Write - Multiple DUTs - Common Data.vi"("Data Out"=w678, "error in"=w665, "Log (T)"=FALSE) -> ("error out"=w673:errorcluster)  [unwired: 12 in]
                    n155 = local write "STATUS"(w674) -> ()
                    n156 = call "Delay.vi"("milliseconds to wait"=u32 10, "error in (no error)"=w673) -> ("error out"=w669:errorcluster)  [unwired: 9 in]
                    n157 = call "WS1050 AD7747 READ 36 DUT.vi"("error in"=w669, "Log (T)"=FALSE, "DUT Mask Mode (All)"=WSVCAP_SHL_I2C_DUT_Mask_Mode_Enum."C3") -> ("error out"=w671:errorcluster, "AD7747 Values"=w670:string[][])  [unwired: 7 in]
                    n158 = for {
                      tunnel: [w685] -> w677 mode=indexing
                      tunnel: w671 -> [w684]
                      tunnel: [w684] -> w667
                      tunnel: w670 -> [w683] mode=indexing
                      n159 = Index Array(array=w683, index=5) -> (element=w685:string)
                    }
                    n160 = Unbundle By Name(w667) -> ("status"=w681:bool)
                    n161 = Or(x=w681, y=w680) -> (x .or. y?=w679:bool)
                  }
                  n162 = Transpose 2D Array(2D array=w601) -> (transposed array=w600:string[][])
                  "VPI C3" <- w600
                }
              }
              n163 = Insert Into Array(array=w536, new element=w506) -> (w535:string[])  [unwired: 1 in]
              n164 = case shown="True" w516 {
                tunnel: w515 -> [w548 w553]
                tunnel: [w549 w552] -> w514
                frame False {
                  n165 = call "WSVCAP SHL Host TL RFFE Write - Multiple DUTs - Common Data.vi"("Data Out"="074820", "error in"=w548, "Log (T)"=FALSE) -> ("error out"=w549:errorcluster)  [unwired: 12 in]
                }
                frame True {
                  n166 = call "WSVCAP SHL Host TL RFFE Write - Multiple DUTs - Common Data.vi"("Data Out"="074800", "error in"=w553, "Log (T)"=FALSE) -> ("error out"=w552:errorcluster)  [unwired: 12 in]
                }
              }
              n167 = call "Delay.vi"("milliseconds to wait"=u32 0, "error in (no error)"=w514) -> ("error out"=w513:errorcluster)  [unwired: 9 in]
            }
            frame #3 {
              # "VSA Testing"
              n168 = case shown="False" w711 {
                tunnel: w749 -> [w761 w775]
                tunnel: [w760 w774] -> w724
                tunnel: [w765 w781] -> w740
                tunnel: w741 -> [w765 w780]
                tunnel: [w762 w778] -> w729
                tunnel: [w762 w777] -> w726
                tunnel: [w762 w776] -> w723
                tunnel: [w763 w779] -> w730
                frame False {
                  n169 = for {
                    tunnel: dbl[] [0.0, 0.0, 0.0] -> [w770] mode=indexing
                    tunnel: [w769] -> w763 mode=indexing
                    tunnel: [w766] -> w762 mode=indexing
                    shift-right: [w767] -> w760
                    shift-left: w761 -> [w767]
                    n170 = Number To Fractional String(number=w770) -> (F-format string=w771:string)  [unwired: 3 in]
                    n171 = for {
                      N: 36 -> [_]
                      tunnel: w771 -> [w773]
                      tunnel: [w773] -> w769 mode=indexing
                      tunnel: [""] -> w766 mode=indexing
                    }
                  }
                }
                frame True {
                  n172 = for {
                    tunnel: "VSA Voltage(V)" -> [w805] mode=indexing
                    tunnel: [w809] -> w781
                    tunnel: w780 -> [w807]
                    tunnel: [w806] -> w778 mode=indexing
                    tunnel: [w793] -> w777 mode=indexing
                    tunnel: [w802] -> w779 mode=indexing
                    tunnel: [w787] -> w776 mode=indexing
                    tunnel: w775 -> [w786]
                    tunnel: [w785] -> w774
                    w784 = FALSE ("Log (T)")
                    w801 = u16 0 items=["Voltage", "Current"] ("Source Mode  (0: Voltage)")
                    n173 = call "Ke2400 Configure Output.vi"("Source Mode  (0: Voltage)"=w801, "error in (no error)"=w786, "Compliance  Level (0.1)"=0.1, "Output Level (0)"=w805, "VISA resource name"=w807) -> ("error out"=w813:errorcluster, "VISA resource name out"=w811:refnum<visa-resource-name>)  [unwired: 5 in]
                    n174 = call "Ke2400 Enable.vi"("error in (no error)"=w813, "ON/OFF"=TRUE ("Enable Output (T: Enable)"), "VISA resource name"=w811) -> ("error out"=w814:errorcluster, "VISA resource name out"=w809:refnum<visa-resource-name>)  [unwired: 7 in]
                    n175 = call "Delay.vi"("milliseconds to wait"=u32 10, "error in (no error)"=w814) -> ("error out"=w800:errorcluster)  [unwired: 9 in]
                    n176 = call "WS1050 AD7747 READ 36 DUT.vi"("error in"=w800, "Log (T)"=w784, "DUT Mask Mode (All)"=WSVCAP_SHL_I2C_DUT_Mask_Mode_Enum."C1") -> ("error out"=w797:errorcluster, "AD7747 Values"=w799:string[][])  [unwired: 7 in]
                    n177 = for {
                      tunnel: w799 -> [w825] mode=indexing
                      tunnel: [w826] -> w806 mode=indexing
                      tunnel: w797 -> [w824]
                      tunnel: [w824] -> w796
                      n178 = Index Array(array=w825, index=1) -> (element=w826:string)
                    }
                    n179 = call "WS1050 AD7747 READ 36 DUT.vi"("error in"=w796, "Log (T)"=w784, "DUT Mask Mode (All)"=WSVCAP_SHL_I2C_DUT_Mask_Mode_Enum."C2") -> ("error out"=w794:errorcluster, "AD7747 Values"=w792:string[][])  [unwired: 7 in]
                    n180 = for {
                      tunnel: w792 -> [w820] mode=indexing
                      tunnel: [w821] -> w793 mode=indexing
                      tunnel: w794 -> [w819]
                      tunnel: [w819] -> w791
                      n181 = Index Array(array=w820, index=3) -> (element=w821:string)
                    }
                    n182 = Number To Fractional String(number=w805) -> (F-format string=w804:string)  [unwired: 3 in]
                    n183 = call "WS1050 AD7747 READ 36 DUT.vi"("error in"=w791, "Log (T)"=w784, "DUT Mask Mode (All)"=WSVCAP_SHL_I2C_DUT_Mask_Mode_Enum."C3") -> ("error out"=w789:errorcluster, "AD7747 Values"=w788:string[][])  [unwired: 7 in]
                    n184 = for {
                      tunnel: w788 -> [w816] mode=indexing
                      tunnel: [w817] -> w787 mode=indexing
                      tunnel: w789 -> [w815]
                      tunnel: [w815] -> w785
                      n185 = Index Array(array=w816, index=5) -> (element=w817:string)
                    }
                    n186 = for {
                      N: 36 -> [_]
                      tunnel: w804 -> [w823]
                      tunnel: [w823] -> w802 mode=indexing
                    }
                  }
                  n187 = local write "STATUS"("VSA Testing...." ("STATUS")) -> ()
                }
              }
              n188 = Transpose 2D Array(2D array=w730) -> (transposed array=w728:string[][])
              n189 = Transpose 2D Array(2D array=w729) -> (transposed array=w727:string[][])
              n190 = Transpose 2D Array(2D array=w726) -> (transposed array=w725:string[][])
              n191 = Transpose 2D Array(2D array=w723) -> (transposed array=w722:string[][])
              n192 = call "WS1050_VSA_Convert_Data.vi"("VSA_C3"=w722, "error in (no error)"=w724, "VSA_C2"=w725, "VSA_C1"=w727, "Voltage"=w728) -> ("error out"=w721:errorcluster, "VSA_V3"=w718:string[][], "VSA_V2"=w719:string[][], "VSA_V1"=w720:string[][])  [unwired: 3 in]
              "VSA_V1" <- w720
              "VSA_V2" <- w719
              "VSA_V3" <- w718
              n193 = case shown="True" w711 {
                tunnel: w740 -> [w753 w759]
                tunnel: [w753 w758] -> w739
                tunnel: w721 -> [w752 w757]
                tunnel: [w752 w754] -> w738
                frame False {
                }
                frame True {
                  w755 = u16 0 items=["Voltage", "Current"] ("Source Mode  (0: Voltage)")
                  n194 = call "Ke2400 Configure Output.vi"("Source Mode  (0: Voltage)"=w755, "error in (no error)"=w757, "Output Level (0)"=0.0, "VISA resource name"=w759) -> ("error out"=w754:errorcluster, "VISA resource name out"=w758:refnum<visa-resource-name>)  [unwired: 6 in]
                }
              }
              n195 = call "Delay.vi"("milliseconds to wait"=u32 0, "error in (no error)"=w738) -> ("error out"=w737:errorcluster)  [unwired: 9 in]
            }
            frame #4 {
              # "Handshake Check and EFuse Readback"
              n196 = Or(x=w839, y=w845) -> (x .or. y?=w844:bool)
              n197 = case shown="True" w844 {
                tunnel: w867 -> [w880 _]
                tunnel: w866 -> [w879 w884]
                tunnel: [w878 w883] -> w865
                tunnel: w864 -> [w877 _]
                tunnel: w863 -> [w876 _]
                tunnel: w862 -> [w875 _]
                tunnel: [w871 w886] -> w861
                tunnel: [w870 w886] -> w856
                tunnel: w829 -> [w869 _]
                tunnel: w850 -> [w868 _]
                frame False {
                  n198 = call "WS1050_36DUT_Handshake Check R1_Record All Regs Ver1.0.vi"("file path (use dialog)"=w880, "Reg1_Bit Cntrl"="Reg1_Bit Cntrl", "File Name"=w868, "SN"=w875, "Loop"=w869, "error"=w879, "Lot #"=w877, "Wafer #"=w876) -> ("Pass/Fail"=→"EFuse Readback Status":bool[], "EFuse Read back"=w870:string[], "Status"=w871:string[], "error out"=w878:errorcluster)  [unwired: 6 in, 2 out]
                  n199 = case shown="1, Default" w869 {
                    tunnel: w870 -> [w881 w882]
                    frame 0 {
                      "EFuse RB T0" <- w881
                    }
                    frame 1, Default {
                      "Current EFuse Read back" <- w882
                    }
                  }
                  n200 = local write "STATUS"("Hand Shake & EFuse Readback...." ("STATUS")) -> ()
                }
                frame True {
                  n201 = for {
                    N: 36 -> [_]
                    tunnel: [""] -> w886 mode=indexing
                    tunnel: w884 -> [w887]
                    tunnel: [w887] -> w883
                  }
                }
              }
              n202 = Build Array(w854, w852, w851) -> (w853:string[])
            }
            frame #5 {
              # "Save Data"
              n203 = Increment(x=w902) -> (x+1=w890:i32)
              n204 = local write "STATUS"("Saving Data...." ("STATUS")) -> ()
              n205 = Multiply(x=w890, y=36) -> (x*y=w898:i32)
              n206 = Path To String(path=w906) -> (string=w905:string)
              n207 = Bundle("Test Program"=w934, "Comment"=w933, "Data Out"=w913, "Data Out"=w912, "CP Voltage"=w911, w910, "% Duty Cycle"=w909, "CP Voltage"=w908, "string"=w907, "Freq(Hz)"=w896, "Board#"=w894) -> (w895:T5)  [unwired: 1 in]
              n208 = case shown="True" w891 {
                tunnel: w898 -> [w941 w944]
                tunnel: [w941 w942] -> w897
                frame False {
                }
                frame True {
                  n209 = Multiply(x=w944, y="No of Rows\nFrom Spread Sheet") -> (x*y=w942:i32)
                }
              }
              n210 = call "WS1050_36 DUT SData Ver1.0.vi"("TMN DC\\CAP Data Log File Path"=w906, "Lot#"=w936, "Total Delta C1(pF)"=w916, "VSA_V1"=w923, "Wafer#"=w932, "File Name"=w900, "Total Delta C2(pF)"=w915, "error in"=w939, "TP/Comment"=w895, "EFuse"=w926, "Data Output C3"=w917, "Temperature"=w921, "VSA_V2"=w924, "VPI C3"=w919, "Data Output C1"=w929, "VPI C2"=w918, "SN"=w937, "R/W Status"=w935, "Cap Header"=w920, "HD/Cycles Completed"="HD/Cycles Completed", "Data Output C2"=w889, "VSA_V3"=w922, "Current"=w928, "VPI C1"=w927, "Total Delta C3(pF)"=w914) -> ("error out"=w938:errorcluster)  [unwired: 2 in]
              n211 = Concatenate Strings(w905, "\\" ("string"), w900, "_Multi Socket Data.csv" ("string")) -> (w904:string)
            }
            frame #6 {
              n212 = case shown="True" "Plot Delta Cmin" {
                tunnel: w952 -> [w961 w976]
                tunnel: [w961 w972] -> w951
                tunnel: w950 -> [_ w968]
                tunnel: w948 -> [_ w966]
                frame False {
                }
                frame True {
                  n213 = String To Path(string=w968) -> (path=w967:path)
                  n214 = call "Delay.vi"("milliseconds to wait"=u32 50, "error in (no error)"=w976) -> ("error out"=w975:errorcluster)  [unwired: 9 in]
                  n215 = call "36DUT Plot From Spread Sheet.vi"("Plot"="Plot", "No of Rows"=w966, "error in (no error)"=w975, "Bank"="Bank1", "file path (dialog if empty)"=w967) -> ("error out"=w970:errorcluster, "Delta C_Min Plot"=→"Plot_1":dbl[][])  [unwired: 5 in]
                  n216 = call "36DUT Plot From Spread Sheet.vi"("Plot"="Plot", "No of Rows"=w966, "error in (no error)"=w970, "Bank"="Bank2", "file path (dialog if empty)"=w967) -> ("error out"=w971:errorcluster, "Delta C_Min Plot"=→"Plot_2":dbl[][])  [unwired: 5 in]
                  n217 = call "36DUT Plot From Spread Sheet.vi"("Plot"="Plot", "No of Rows"=w966, "error in (no error)"=w971, "Bank"="Bank3", "file path (dialog if empty)"=w967) -> ("error out"=w972:errorcluster, "Delta C_Min Plot"=→"Plot_3":dbl[][])  [unwired: 5 in]
                }
              }
              n218 = Increment(x=w946) -> (x+1=w945:i32)
              "No of HD/Cycle\nCompleted" <- w945
              n219 = Get Date/Time In Seconds() -> (seconds since 1Jan1904=w954:timestamp)
              n220 = Get Date/Time String(seconds (now)=w954, want seconds? (F)=TRUE) -> (date string=→"date string":string, time string=→"Previous Time":string)  [unwired: 1 in]
              n221 = Greater Or Equal?(x=w945, y=w947) -> (x >= y?=w958:bool)
            }
          }
          n222 = Compound Arithmetic op=OR(w308, w228) -> (w257:bool)
          n223 = call "Delay.vi"("milliseconds to wait"=u32 10, "error in (no error)"=w193) -> ("error out"=w194:errorcluster)  [unwired: 9 in]
          "Loop \ncompleted" <- w156
        }
        n224 = local write "No of HD/Cycle\nCompleted"(u64 0 ("No of HD/Cycle\nCompleted")) -> ()
      }
      n225 = VISA Write(VISA resource name=w59, write buffer="SOUR:FUNC VOLT;VOLT:MODE FIX;RANG 100;LEV 0.0;:SENS:FUNC \"CURR\";CURR:PROT 60E-3;RANG 100E-3;:OUTP ON", error in (no error)=w50) -> (VISA resource name out=w58:refnum<visa-resource-name>, error out=w34:errorcluster)  [unwired: 1 out]
    }
  }
  "Ke2000 Out" <- w22
  "PS1 Out" <- w21
  "Ke2400 Out" <- w16
  "error out" <- w15
  "STATUS" <- "Idle...." ("STATUS")
